vi "Update UI.vi"(8 "error in (no error)":errorcluster, 11 "Message Logger in":refnum<class "Classic Logger.lvclass">) -> (0 "error out":errorcluster, 3 "Message Logger out":refnum<class "Classic Logger.lvclass">)   [LabVIEW 2023, in "Monitored Actor.lvlib" / "Classic Logger.lvclass"]
doc: "Builds the data to update the UI\n\nCopyright: MGI 2016\nAuthor: Derek Trepanier"
uses:
  Classic Logger.lvclass
  UI Data.ctl
  builds/Engine/Actor Framework.lvlibp/1abvi3w/vi.lib/ActorFramework/Message Enqueuer/Message Enqueuer.lvclass
  Classic Logger.lvclass/Classic Logger.ctl
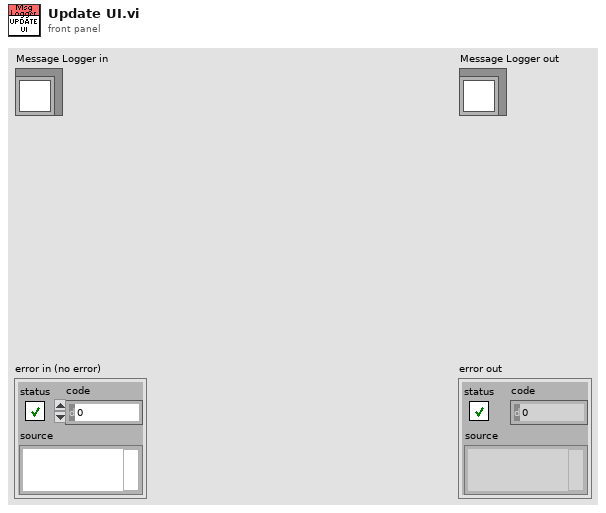
[diagram p1: front panel]
types:
  T1 = typedef "Monitored Actor.lvlib/Classic Logger.lvclass/UI Data.ctl" = cluster{"Actors":cluster{"Q":refnum<class "Message Enqueuer.lvclass">, "Label":string}[], "Message Log":variant}
  T2 = cluster{"Q":refnum<class "Message Enqueuer.lvclass">, "data string":string}
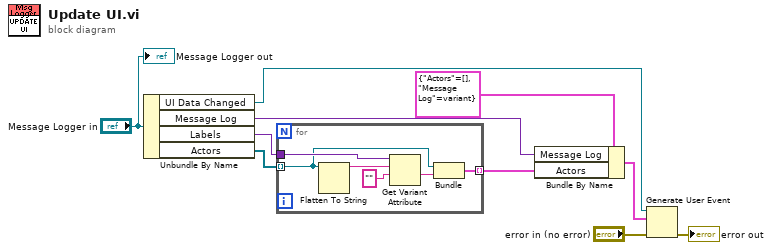
[diagram p0: block diagram]
diagram:
  n1 = Unbundle By Name("Message Logger in") -> ("UI Data Changed"=w7:refnum<user-event>, "Message Log"=w5:variant, "Labels"=w3:variant, "Actors"=w4:refnum<class "Message Enqueuer.lvclass">[])
  n2 = for {
    tunnel: w4 -> [w13] mode=indexing
    tunnel: w3 -> [w16]
    tunnel: [w11] -> w2 mode=indexing
    n3 = Flatten To String(anything=w13) -> (data string=w15:string)  [unwired: 3 in, 2 out]
    n4 = Get Variant Attribute(Variant=w16, name=w15, default value (empty Variant)="" ("data string")) -> (value=w12:string)  [unwired: 1 in, 3 out]
    n5 = Bundle("Q"=w13, "data string"=w12) -> (w11:T2)  [unwired: 1 in]
  }
  n6 = Bundle By Name(cluster=T1 {"Actors"=[], "Message Log"=variant} ("UI Data"), "Message Log"=w5, "Actors"=w2) -> (w1:T1)
  n7 = Generate User Event(user event=w7, event data cluster=w1, error in="error in (no error)") -> (error out=→"error out":errorcluster)  [unwired: 1 in, 1 out]
  "Message Logger out" <- "Message Logger in"
